vi "Popup.vi"(8 "error in (no error)":errorcluster, 9 "Panel":refnum<class "Panel.lvclass">, 10 "String in":string, 11 "Numeric Data Type in":refnum<class "Numeric Data Type.lvclass">) -> (0 "error out":errorcluster, 2 "String out":string, 3 "Numeric Data Type out":refnum<class "Numeric Data Type.lvclass">)   [LabVIEW 2018, in "Numeric Data Type.lvclass"]
uses:
  Numeric Data Type.lvclass
  <vilib>/MGI/Panel Manager/Panel/Panel/Panel.lvclass
  Numeric Data Type.lvclass/Numeric Data Type.ctl
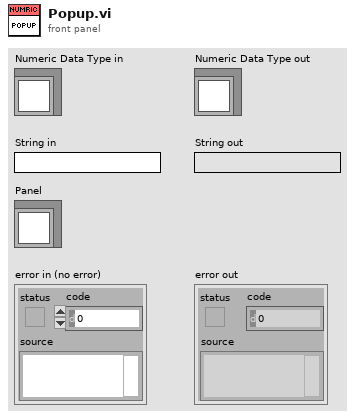
[diagram p1: front panel]
types:
  T1 = typedef "Numeric Data Type.lvclass/Representation Enum.ctl" = enum16{"Extended (EXT)", "Double (DBL)", "Single (SGL)", "Fixed-Point (FXP)", "Quad Integer (I64)", "Long Integer (I32)", "Word Integer (I16)", "Byte Integer (I8)", "Unsigned Quad (U64)", "Unsigned Long (U32)", "Unsigned Word (U16)", "Unsigned Byte (U8)", "Complex Extended (CXT)", "Complex Double (CDB)", "Complex Single (CSG)"}
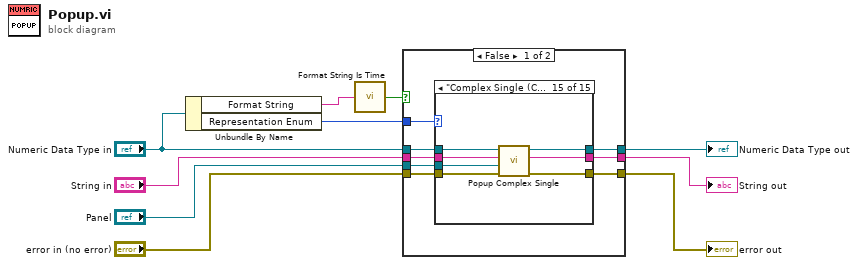
[diagram p0: block diagram]
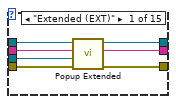
[diagram p2: hidden frame]
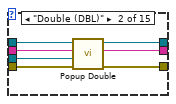
[diagram p3: hidden frame]
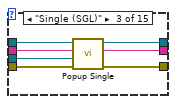
[diagram p4: hidden frame]
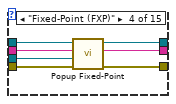
[diagram p5: hidden frame]
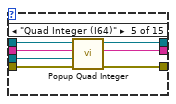
[diagram p6: hidden frame]
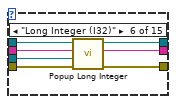
[diagram p7: hidden frame]
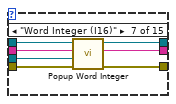
[diagram p8: hidden frame]
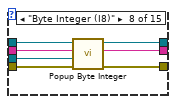
[diagram p9: hidden frame]
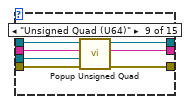
[diagram p10: hidden frame]
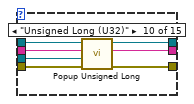
[diagram p11: hidden frame]
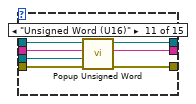
[diagram p12: hidden frame]
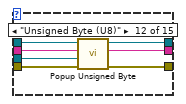
[diagram p13: hidden frame]
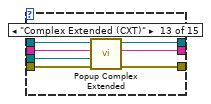
[diagram p14: hidden frame]
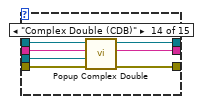
[diagram p15: hidden frame]
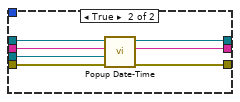
[diagram p16: hidden frame]
diagram:
  n1 = Unbundle By Name("Numeric Data Type in") -> ("Format String"=w2:string, "Representation Enum"=w10:T1)
  n2 = call "Format String Is Time.vi"("Format String"=w2) -> ("Time?"=w1:bool)
  n3 = case shown="False" w1 {
    tunnel: w10 -> [w18 _]
    tunnel: "Numeric Data Type in" -> [w17 w130]
    tunnel: [w16 w129] -> w8
    tunnel: "String in" -> [w15 w128]
    tunnel: "Panel" -> [w14 w127]
    tunnel: [w13 w126] -> w5
    tunnel: "error in (no error)" -> [w12 w125]
    tunnel: [w11 w124] -> w3
    frame False {
      n4 = case shown="\"Complex Single (CSG)\"" w18 {
        tunnel: w17 -> [w25 w32 w39 w46 w53 w60 w67 w74 w81 w88 w95 w102 w109 w116 w123]
        tunnel: [w24 w31 w38 w44 w52 w59 w63 w70 w77 w84 w94 w98 w105 w112 w119] -> w16
        tunnel: w15 -> [w23 w29 w37 w45 w51 w58 w66 w73 w80 w87 w93 w101 w108 w115 w122]
        tunnel: w14 -> [w22 w28 w35 w42 w49 w56 w65 w72 w79 w86 w91 w100 w107 w114 w121]
        tunnel: [w21 w30 w36 w43 w50 w57 w62 w69 w76 w83 w92 w97 w104 w111 w118] -> w13
        tunnel: w12 -> [w20 w26 w34 w41 w48 w55 w64 w71 w78 w85 w90 w99 w106 w113 w120]
        tunnel: [w19 w27 w33 w40 w47 w54 w61 w68 w75 w82 w89 w96 w103 w110 w117] -> w11
        frame "Extended (EXT)" {
          n5 = call "Popup Extended.vi"("error in (no error)"=w20, "Panel"=w22, "String in"=w23, "Numeric Data Type in"=w25) -> ("error out"=w19:errorcluster, "String out"=w21:string, "Numeric Data Type out"=w24:refnum<class "Numeric Data Type.lvclass">)  [unwired: 5 in]
        }
        frame "Double (DBL)" {
          n6 = call "Popup Double.vi"("error in (no error)"=w26, "Panel"=w28, "String in"=w29, "Numeric Data Type in"=w32) -> ("error out"=w27:errorcluster, "String out"=w30:string, "Numeric Data Type out"=w31:refnum<class "Numeric Data Type.lvclass">)  [unwired: 5 in]
        }
        frame "Single (SGL)" {
          n7 = call "Popup Single.vi"("error in (no error)"=w34, "Panel"=w35, "String in"=w37, "Numeric Data Type in"=w39) -> ("error out"=w33:errorcluster, "String out"=w36:string, "Numeric Data Type out"=w38:refnum<class "Numeric Data Type.lvclass">)  [unwired: 5 in]
        }
        frame "Fixed-Point (FXP)" {
          n8 = call "Popup Fixed-Point.vi"("error in (no error)"=w41, "Panel"=w42, "String in"=w45, "Numeric Data Type in"=w46) -> ("error out"=w40:errorcluster, "String out"=w43:string, "Numeric Data Type out"=w44:refnum<class "Numeric Data Type.lvclass">)  [unwired: 5 in]
        }
        frame "Quad Integer (I64)" {
          n9 = call "Popup Quad Integer.vi"("error in (no error)"=w48, "Panel"=w49, "String in"=w51, "Numeric Data Type in"=w53) -> ("error out"=w47:errorcluster, "String out"=w50:string, "Numeric Data Type out"=w52:refnum<class "Numeric Data Type.lvclass">)  [unwired: 5 in]
        }
        frame "Long Integer (I32)" {
          n10 = call "Popup Long Integer.vi"("error in (no error)"=w55, "Panel"=w56, "String in"=w58, "Numeric Data Type in"=w60) -> ("error out"=w54:errorcluster, "String out"=w57:string, "Numeric Data Type out"=w59:refnum<class "Numeric Data Type.lvclass">)  [unwired: 5 in]
        }
        frame "Word Integer (I16)" {
          n11 = call "Popup Word Integer.vi"("error in (no error)"=w64, "Panel"=w65, "String in"=w66, "Numeric Data Type in"=w67) -> ("error out"=w61:errorcluster, "String out"=w62:string, "Numeric Data Type out"=w63:refnum<class "Numeric Data Type.lvclass">)  [unwired: 5 in]
        }
        frame "Byte Integer (I8)" {
          n12 = call "Popup Byte Integer.vi"("error in (no error)"=w71, "Panel"=w72, "String in"=w73, "Numeric Data Type in"=w74) -> ("error out"=w68:errorcluster, "String out"=w69:string, "Numeric Data Type out"=w70:refnum<class "Numeric Data Type.lvclass">)  [unwired: 5 in]
        }
        frame "Unsigned Quad (U64)" {
          n13 = call "Popup Unsigned Quad.vi"("error in (no error)"=w78, "Panel"=w79, "String in"=w80, "Numeric Data Type in"=w81) -> ("error out"=w75:errorcluster, "String out"=w76:string, "Numeric Data Type out"=w77:refnum<class "Numeric Data Type.lvclass">)  [unwired: 5 in]
        }
        frame "Unsigned Long (U32)" {
          n14 = call "Popup Unsigned Long.vi"("error in (no error)"=w85, "Panel"=w86, "String in"=w87, "Numeric Data Type in"=w88) -> ("error out"=w82:errorcluster, "String out"=w83:string, "Numeric Data Type out"=w84:refnum<class "Numeric Data Type.lvclass">)  [unwired: 5 in]
        }
        frame "Unsigned Word (U16)" {
          n15 = call "Popup Unsigned Word.vi"("error in (no error)"=w90, "Panel"=w91, "String in"=w93, "Numeric Data Type in"=w95) -> ("error out"=w89:errorcluster, "String out"=w92:string, "Numeric Data Type out"=w94:refnum<class "Numeric Data Type.lvclass">)  [unwired: 5 in]
        }
        frame "Unsigned Byte (U8)" {
          n16 = call "Popup Unsigned Byte.vi"("error in (no error)"=w99, "Panel"=w100, "String in"=w101, "Numeric Data Type in"=w102) -> ("error out"=w96:errorcluster, "String out"=w97:string, "Numeric Data Type out"=w98:refnum<class "Numeric Data Type.lvclass">)  [unwired: 5 in]
        }
        frame "Complex Extended (CXT)" {
          n17 = call "Popup Complex Extended.vi"("error in (no error)"=w106, "Panel"=w107, "String in"=w108, "Numeric Data Type in"=w109) -> ("error out"=w103:errorcluster, "String out"=w104:string, "Numeric Data Type out"=w105:refnum<class "Numeric Data Type.lvclass">)  [unwired: 5 in]
        }
        frame "Complex Double (CDB)" {
          n18 = call "Popup Complex Double.vi"("error in (no error)"=w113, "Panel"=w114, "String in"=w115, "Numeric Data Type in"=w116) -> ("error out"=w110:errorcluster, "String out"=w111:string, "Numeric Data Type out"=w112:refnum<class "Numeric Data Type.lvclass">)  [unwired: 5 in]
        }
        frame "Complex Single (CSG)" {
          n19 = call "Popup Complex Single.vi"("error in (no error)"=w120, "Panel"=w121, "String in"=w122, "Numeric Data Type in"=w123) -> ("error out"=w117:errorcluster, "String out"=w118:string, "Numeric Data Type out"=w119:refnum<class "Numeric Data Type.lvclass">)  [unwired: 5 in]
        }
      }
    }
    frame True {
      n20 = call "Popup Date-Time.vi"("error in (no error)"=w125, "Panel"=w127, "String in"=w128, "Numeric Data Type in"=w130) -> ("error out"=w124:errorcluster, "String out"=w126:string, "Numeric Data Type out"=w129:refnum<class "Numeric Data Type.lvclass">)  [unwired: 5 in]
    }
  }
  "error out" <- w3
  "Numeric Data Type out" <- w8
  "String out" <- w5
